vi "validation_caoo.vi"() -> ()   [LabVIEW 2024]
uses:
  <vilib>/addons/control/pid/pid.llb/PID Structure.ctl
  <vilib>/addons/control/pid/pid.llb/PID Time Unit.ctl
  <vilib>/addons/control/pid/pid.llb/PID Gain Unit.ctl
  <vilib>/addons/control/pid/pid.llb/PID Structure Conversion (DBL).vi
  <vilib>/addons/control/pid/pid.llb/PID Advanced (DBL).vi
  <vilib>/ptbypt/NI_PtbyPt.lvlib
  <vilib>/addons/control/pid/NI_PID_pid.lvlib
panel:
  in  "u1":dbl(slide) scale=0.0..100.0
  in  "Manual 3":bool
  in  "u2":dbl(slide) scale=0.0..100.0
  in  "Manual 2":bool
  out "Waveform Chart 2":cluster{"Setpoint":dbl, "Centimeters":dbl}(graph)
  out "Waveform Chart":cluster{"Setpoint":dbl, "Centimeters":dbl}(graph)
  in  "Initialize 2":bool caption="Initialize"
  out "PID (dt) 4":dbl
  in  "PID (dt)  3":dbl
  out "PID2 output 2":dbl format="%.1f"
  out "PID1 output":dbl format="%.1f"
  out "hre2":dbl(slide) scale=0.0..16.0
  in  "hre2":dbl
  out "hre1":dbl(slide) scale=0.0..16.0
  in  "hre1":dbl
  in  "stop":bool
  in  "output_h  range":cluster{"output high":dbl, "output low":dbl}={"output high"=60.0, "output low"=0.0} {"output high" min=0.0 max=60.0 format="%.2f"; "output low" min=0.0 max=60.0 format="%.2f"}
  in  "Proportional Unit":T1 items=["Gain (Kc)", "Band (PB)"]
  in  "Derivative Unit":T2 items=["min", "s"]
  in  "Integral Unit":T2 items=["min", "s"]
  in  "PID Topology":T3 items=["Academic (Standard)", "Parallel", "Series"]
  in  "Derivative":dbl format="%#.3g"
  in  "Integral":dbl=0.008 format="%#.3g"
  in  "Proportional":dbl=5.0 format="%#.10f"
  in  "Initialize":bool
  in  "setpoint_href range":cluster{"setpoint high":dbl, "setpoint low":dbl}={"setpoint high"=60.0, "setpoint low"=0.0} {"setpoint high" min=0.0 max=60.0 format="%.2f"; "setpoint low" min=0.0 max=60.0 format="%.2f"}
  in  "a":dbl
  out "PID (dt) 2":dbl
  in  "PID (dt)":dbl
  out "Q20":dbl
  out "Q32":dbl
  out "Q13":dbl
  in  "Sn":dbl
  out "h2":dbl
  out "h3":dbl
  out "h1":dbl
  in  "S":dbl
  out "vh2":dbl
  out "vh3":dbl
  out "vh1":dbl
  out "Tank 3":dbl(slide) scale=0.0..10.0
  out "Tank 2":dbl(slide) scale=0.0..10.0
  out "Tank 1":dbl(slide) scale=0.0..10.0
  # "TT Parameters"
  # "TT Outputs"
  # "Cas ou PID est manuel"
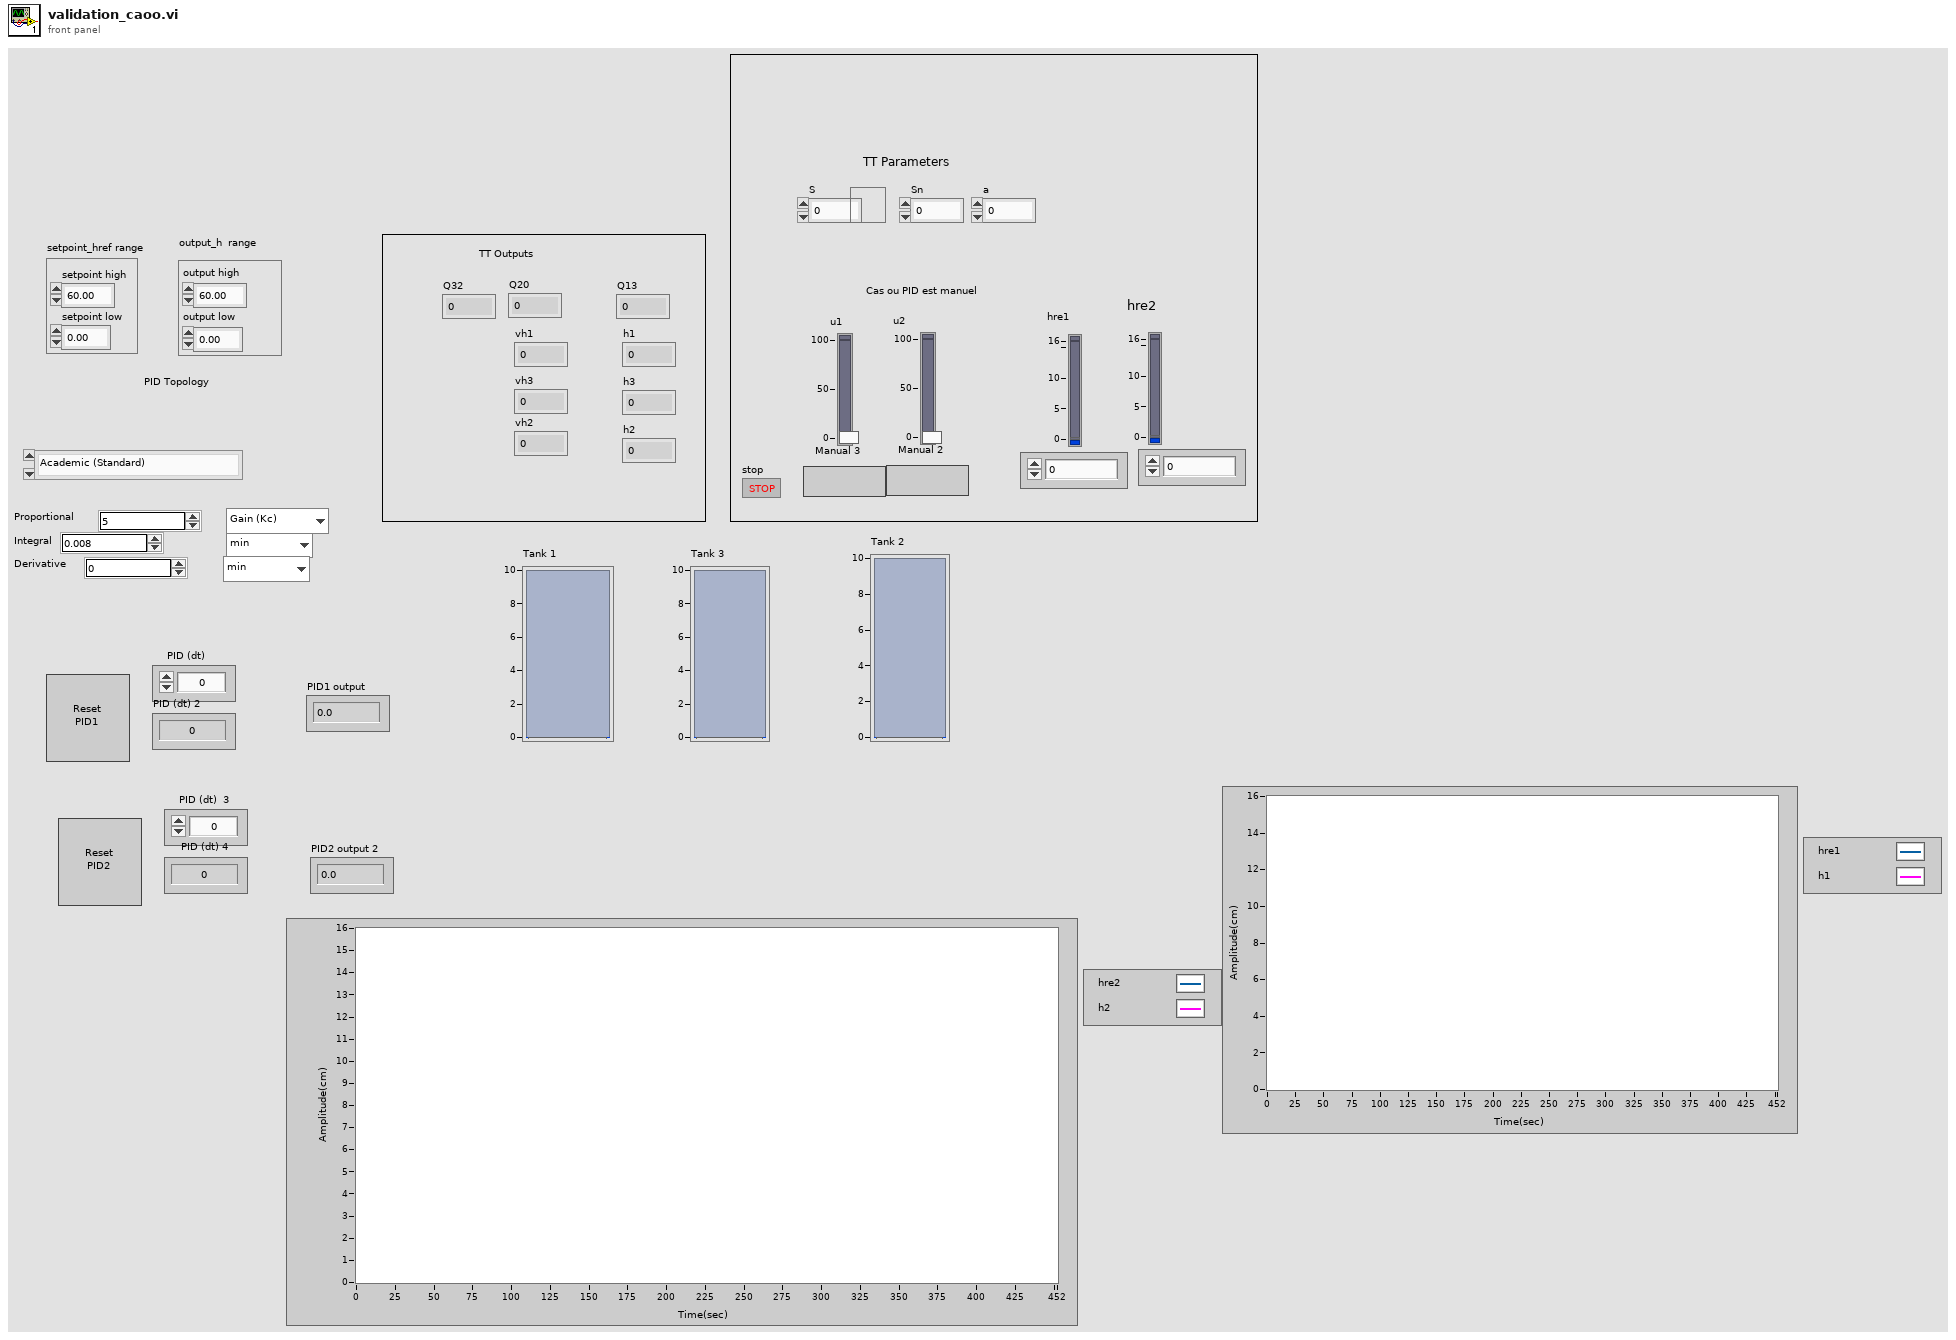
[diagram p1: front panel]
types:
  T1 = typedef "NI_PID_pid.lvlib/PID Gain Unit.ctl" = u16
  T2 = typedef "NI_PID_pid.lvlib/PID Time Unit.ctl" = u16
  T3 = typedef "NI_PID_pid.lvlib/PID Structure.ctl" = u16
  T4 = cluster{"proportional gain (Kc)":dbl, "integral time (Ti, min)":dbl, "derivative time (Td, min)":dbl}
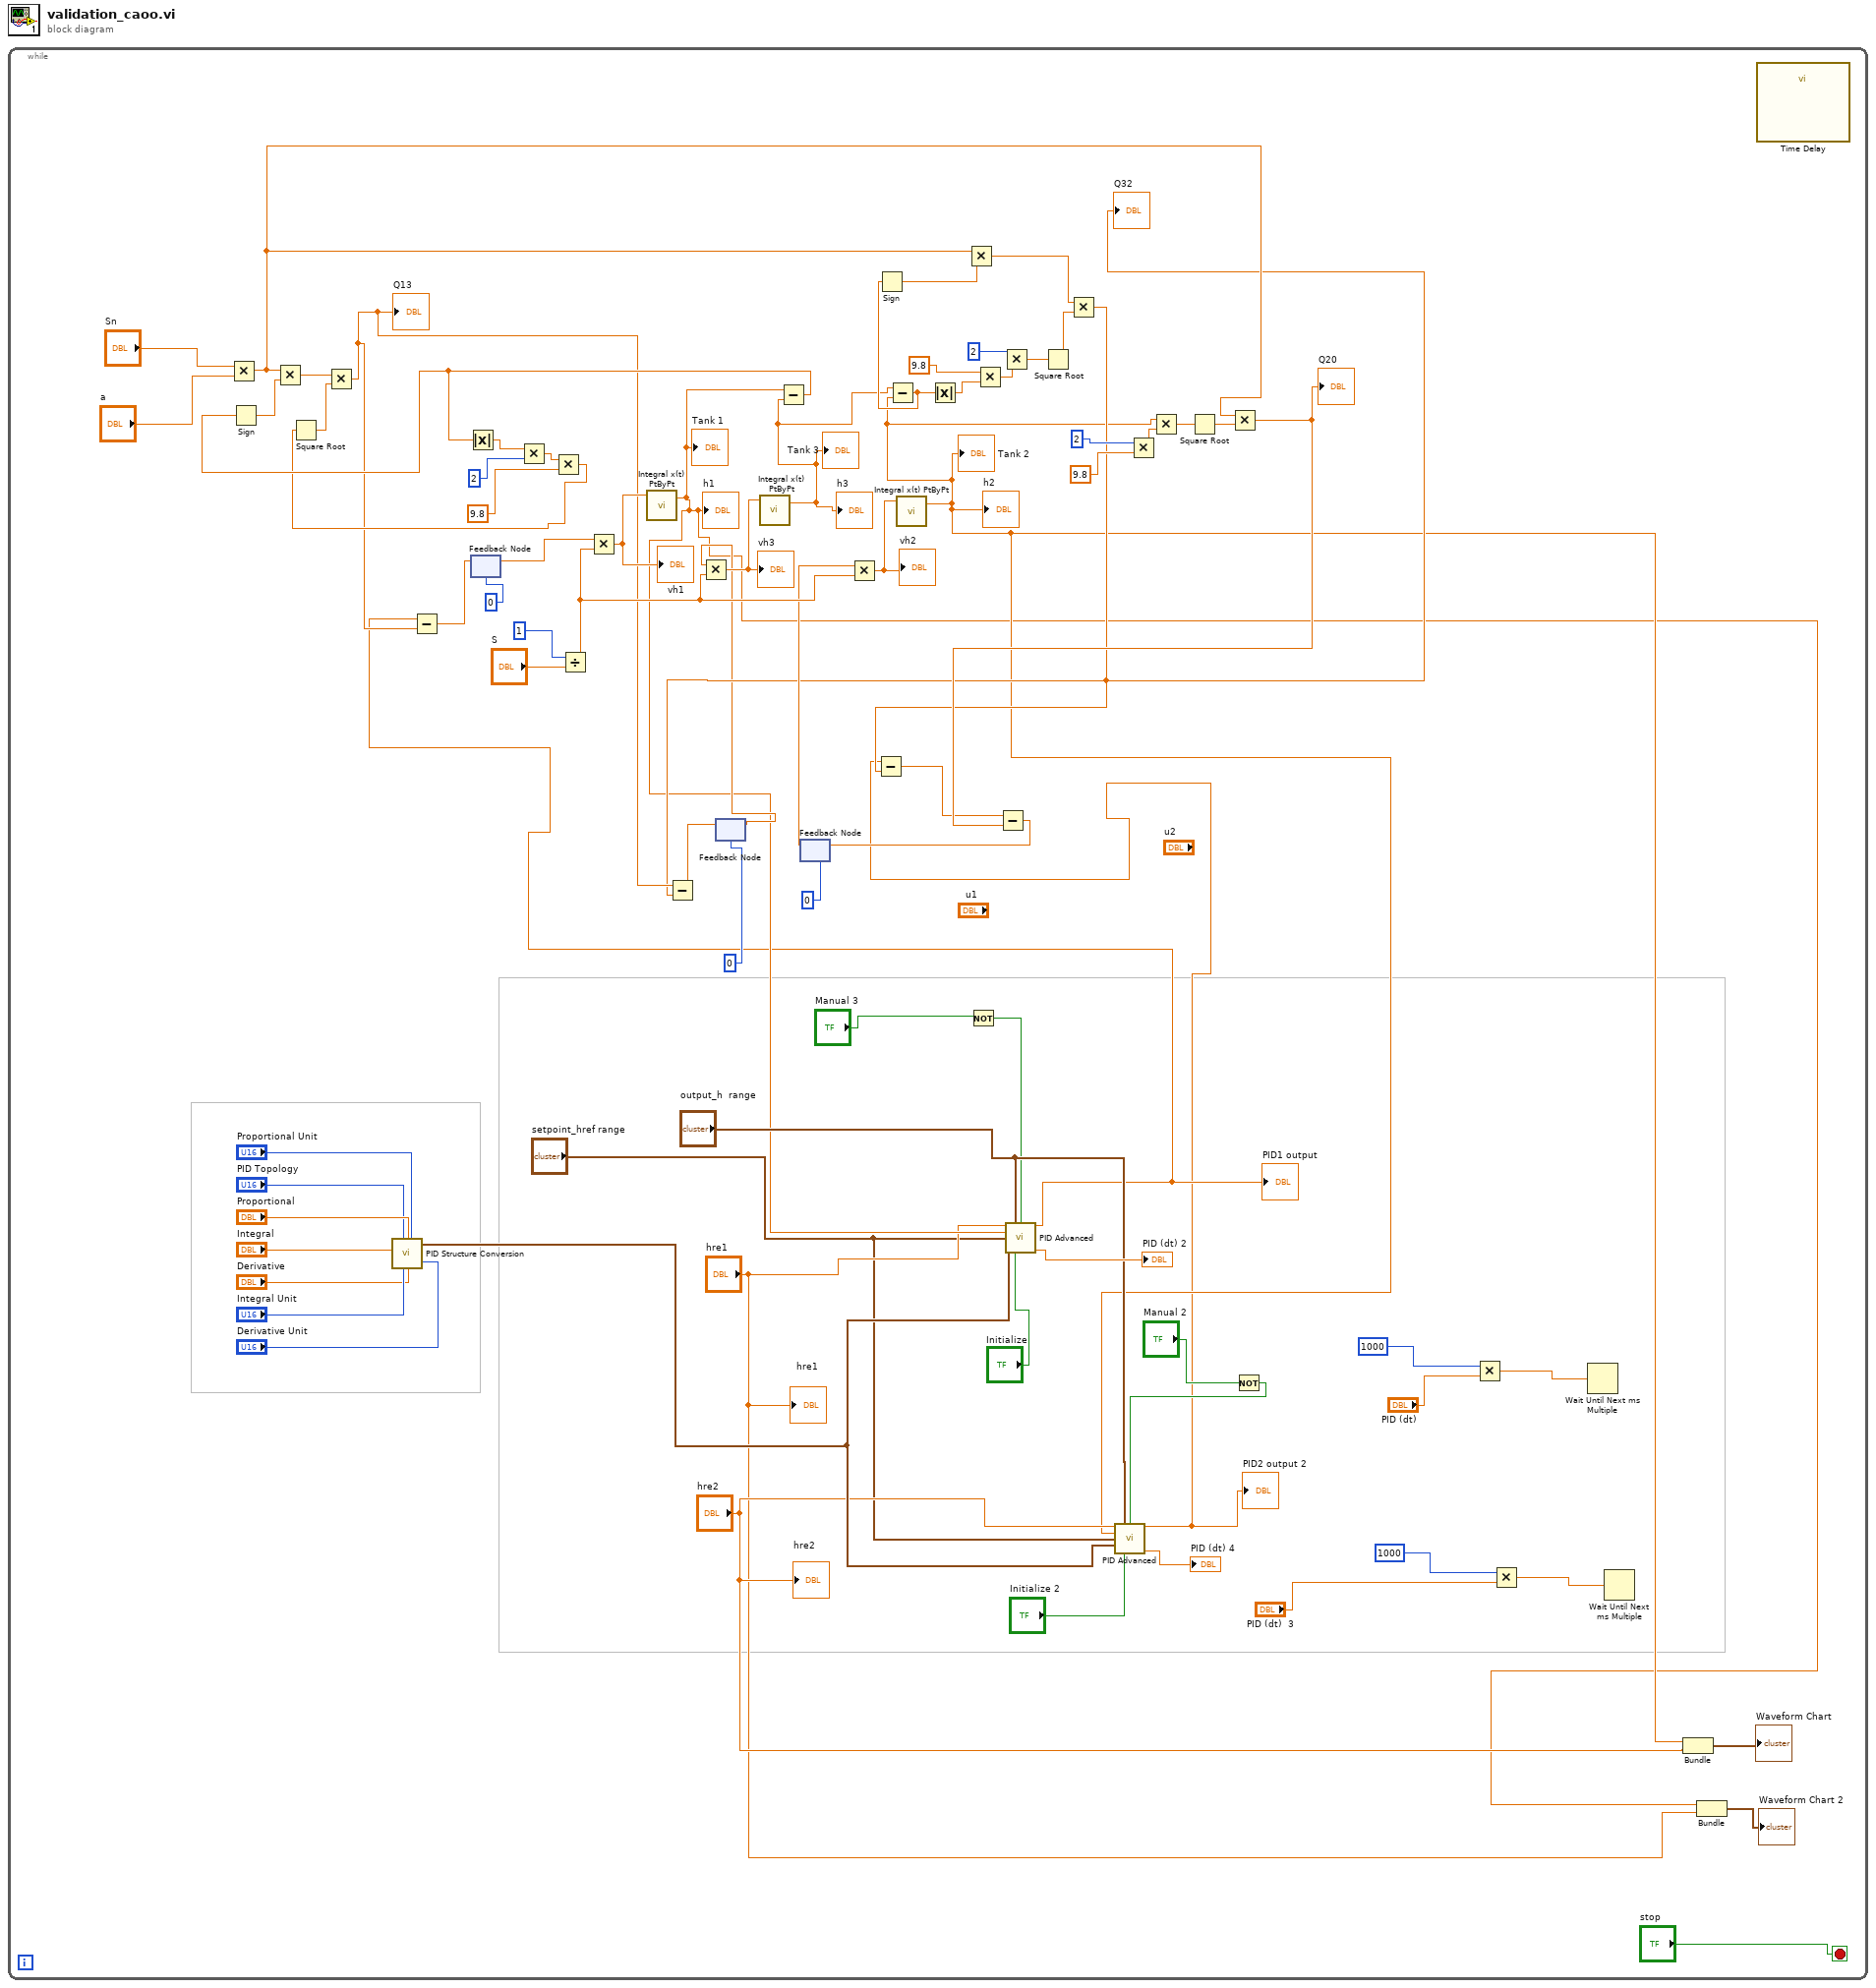
[diagram p0: block diagram]
diagram:
  n1 = while {
    stop <- "stop" stop-if-true
    n2 = Multiply(x="Sn", y="a") -> (x*y=w38:dbl)
    n3 = call-poly <vilib>:"PID Structure Conversion.vi"("derivative unit"="Derivative Unit", "proportional unit"="Proportional Unit", "integral unit"="Integral Unit", "PID structure"="PID Topology", "derivative"="Derivative", "integral"="Integral", "proportional"="Proportional") -> ("PID gains"=w22:T4)  [unwired: 4 in]
    n4 = feedback #1(0) -> (w49:dbl)
    n5 = Divide(x=1, y="S") -> (x/y=w77:dbl)
    n6 = Multiply(x=w49, y=w77) -> (x*y=w76:dbl)
    "vh1" <- w76
    n7 = call <vilib>:"Integral x(t) PtByPt.vi"("x"=w76) -> ("integral x(t)"=w6:dbl)  [unwired: 3 in, 1 out]
    "Tank 1" <- w6
    "h1" <- w6
    n8 = feedback #2(0) -> (w34:dbl)
    n9 = Multiply(x=w34, y=w77) -> (x*y=w75:dbl)
    "vh3" <- w75
    n10 = call <vilib>:"Integral x(t) PtByPt.vi"("x"=w75) -> ("integral x(t)"=w41:dbl)  [unwired: 3 in, 1 out]
    "Tank 3" <- w41
    "h3" <- w41
    n11 = Subtract(x=w6, y=w41) -> (x-y=w70:dbl)
    n12 = Sign(1:w70) -> (0:w73:dbl)
    n13 = Multiply(x=w38, y=w73) -> (x*y=w72:dbl)
    n14 = Absolute Value(x=w70) -> (abs(x)=w69:dbl)
    n15 = Multiply(x=w69, y=2) -> (x*y=w66:dbl)
    n16 = Multiply(x=w66, y=9.8) -> (x*y=w65:dbl)
    n17 = Square Root(x=w65) -> (sqrt(x)=w71:dbl)
    n18 = Multiply(x=w72, y=w71) -> (x*y=w44:dbl)
    "Q13" <- w44
    n19 = feedback #3(0) -> (w45:dbl)
    n20 = Multiply(x=w45, y=w77) -> (x*y=w74:dbl)
    "vh2" <- w74
    n21 = call <vilib>:"Integral x(t) PtByPt.vi"("x"=w74) -> ("integral x(t)"=w12:dbl)  [unwired: 3 in, 1 out]
    "Tank 2" <- w12
    "h2" <- w12
    n22 = Subtract(x=w41, y=w12) -> (x-y=w59:dbl)
    n23 = Sign(1:w59) -> (0:w58:dbl)
    n24 = Absolute Value(x=w59) -> (abs(x)=w64:dbl)
    n25 = Multiply(x=w38, y=w58) -> (x*y=w37:dbl)
    n26 = Not(x="Manual 3") -> (.not. x?=w4:bool)
    n27 = Multiply(x=9.8, y=w64) -> (x*y=w62:dbl)
    n28 = Multiply(x=2, y=w62) -> (x*y=w60:dbl)
    n29 = call-poly <vilib>:"PID Advanced.vi"("setpoint"="hre1", "output range"="output_h  range", "auto? (T)"=w4, "process variable"=w6, "setpoint range"="setpoint_href range", "PID gains"=w22, "reinitialize? (F)"="Initialize") -> ("output"=w2:dbl, "dt out (s)"=→"PID (dt) 2":dbl)  [unwired: 7 in]
    "PID1 output" <- w2
    n30 = Subtract(x=w2, y=w44) -> (x-y=w50:dbl)
    n31 = feedback-in #1(w50) -> ()
    n32 = Square Root(x=w60) -> (sqrt(x)=w57:dbl)
    n33 = Multiply(x=w37, y=w57) -> (x*y=w35:dbl)
    "Q32" <- w35
    n34 = Subtract(x=w44, y=w35) -> (x-y=w43:dbl)
    n35 = feedback-in #2(w43) -> ()
    n36 = Multiply(x=2, y=9.8) -> (x*y=w54:dbl)
    n37 = Multiply(x=w12, y=w54) -> (x*y=w53:dbl)
    n38 = Square Root(x=w53) -> (sqrt(x)=w52:dbl)
    n39 = Multiply(x=w38, y=w52) -> (x*y=w39:dbl)
    "Q20" <- w39
    n40 = Not(x="Manual 2") -> (.not. x?=w9:bool)
    n41 = call-poly <vilib>:"PID Advanced.vi"("setpoint"="hre2", "output range"="output_h  range", "auto? (T)"=w9, "process variable"=w12, "setpoint range"="setpoint_href range", "PID gains"=w22, "reinitialize? (F)"="Initialize 2") -> ("output"=w1:dbl, "dt out (s)"=→"PID (dt) 4":dbl)  [unwired: 7 in]
    "PID2 output 2" <- w1
    n42 = Subtract(x=w1, y=w35) -> (x-y=w36:dbl)
    n43 = Subtract(x=w36, y=w39) -> (x-y=w47:dbl)
    n44 = feedback-in #3(w47) -> ()
    n45 = Multiply(x=1000, y="PID (dt)") -> (x*y=w23:dbl)
    n46 = Multiply(x=1000, y="PID (dt)  3") -> (x*y=w18:dbl)
    n47 = Wait Until Next ms Multiple(millisecond multiple=w23) -> ()  [unwired: 1 out]
    n48 = Wait Until Next ms Multiple(millisecond multiple=w18) -> ()  [unwired: 1 out]
    n49 = Bundle("integral x(t)"=w12, "hre2"="hre2") -> (→"Waveform Chart":cluster{"integral x(t)":dbl, "hre2":dbl})  [unwired: 1 in]
    n50 = Bundle("integral x(t)"=w6, "hre1"="hre1") -> (→"Waveform Chart 2":cluster{"integral x(t)":dbl, "hre1":dbl})  [unwired: 1 in]
    n51 = call "Time Delay"() -> ()  [unwired: 11 in, 1 out]
    "hre1" <- "hre1"
    "hre2" <- "hre2"
  }
